vi "XIPIN_SMPTE_UHD-SDI_1_0.vi"   [LabVIEW 2017]
doc: "SMPTE UHD Serial Digital Interface carries uncompressed digital video and ancillary data and supports data rate from SD-SDI through 12G-SDI\n------------------------------------\n<b>Need License</b> : No"
uses:
  <vilib>/rvi/XilinxIP/XIPIN_XNode/niFpgaXIPIN.xnode
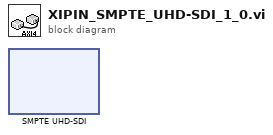
[diagram p0: block diagram]
diagram:
  n1 = xnode ("SMPTE UHD-SDI")() -> ()
